vi "write KPRO file.vi"(9 "Corrected Array in":dbl[][](array[numeric]), 10 "Generate Array Calc IK":bool, 11 "Path in":refnum<vi>) -> (1 "paths ok":bool, 3 "appended path":path)   [LabVIEW 2016]
uses:
  <vilib>/Utility/file.llb/Write Delimited Spreadsheet (DBL).vi
panel:
  out "type":i16
  out "Value":path
  out "error out":errorcluster
  in  "error in (no error)":errorcluster
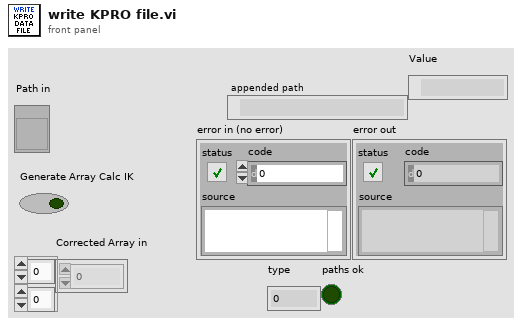
[diagram p1: front panel]
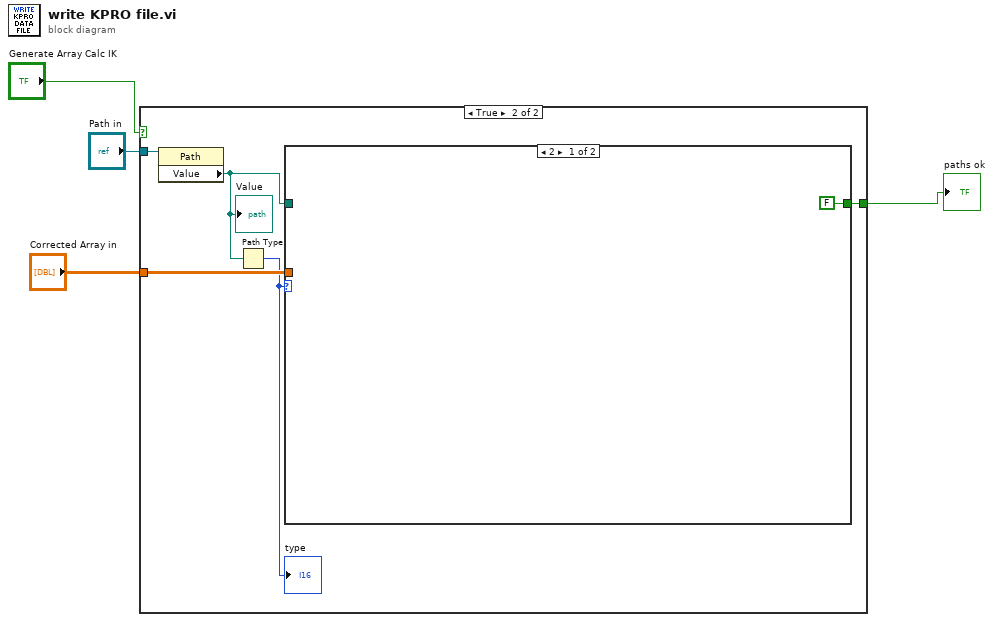
[diagram p0: block diagram]
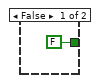
[diagram p2: hidden frame]
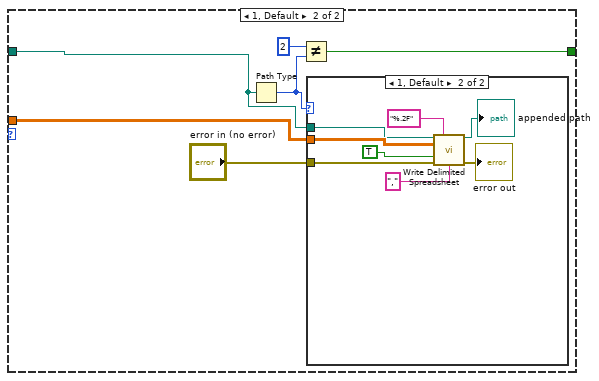
[diagram p3: hidden frame]
diagram:
  n1 = case shown="True" "Generate Array Calc IK" {
    tunnel: "Corrected Array in" -> [_ w10]
    tunnel: "Path in" -> [_ w9]
    tunnel: [FALSE w6] -> w1
    frame False {
    }
    frame True {
      n2 = property class="Path"(reference=w9) -> ("Value"=w8:path)  [unwired: 1 in, 2 out]
      "Value" <- w8
      n3 = Path Type(1:w8) -> (0:w7:i16)
      "type" <- w7
      n4 = case shown="2" w7 {
        tunnel: w10 -> [_ w17]
        tunnel: w8 -> [_ w12]
        tunnel: [FALSE w13] -> w6
        frame 2 {
        }
        frame 1, Default {
          n5 = Path Type(1:w12) -> (0:w15:i16)
          n6 = Not Equal?(x=i16 2, y=w15) -> (x != y?=w13:bool)
          n7 = case shown="1, Default" w15 {
            tunnel: w17 -> [_ w25]
            tunnel: "error in (no error)" -> [_ w21]
            tunnel: w12 -> [_ w19]
            frame 2 {
            }
            frame 1, Default {
              n8 = call-poly <vilib>:"Write Delimited Spreadsheet.vi"("file path (dialog if empty)"=w19, "format (%.3f)"="%.2F", "2D data"=w25, "append to file? (new file:F)"=TRUE, "error in (no error)"=w21, "delimiter (\\t)"="," ("delimiter (\\t)")) -> ("new file path (Not A Path if cancelled)"=→"appended path":path, "error out"=→"error out":errorcluster)  [unwired: 8 in]
            }
          }
        }
      }
    }
  }
  "paths ok" <- w1
